vi "m10.wf.ramp.vi"(0 "Waveform In":waveform(dbl)={"t0"=timestamp(0 s since 1904-01-01), "dt"=0.0, "Y"=[]}, 5 "Ramp Length (s)":dbl=0.01, 11 "error in (no error)":errorcluster) -> (4 "Waveform Out":waveform(dbl), 15 "error out":errorcluster)   [LabVIEW 2013]
uses:
  <vilib>/Waveform/WDTOps.llb/WDT Waveform Duration DBL.vi
  <vilib>/Waveform/WDTOps.llb/WDT Append Waveforms DBL.vi
  <vilib>/measure/NI_MABase.lvlib
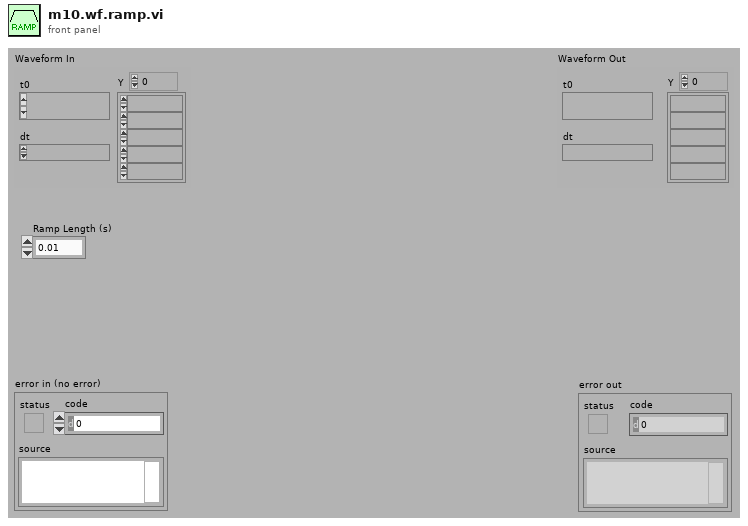
[diagram p1: front panel]
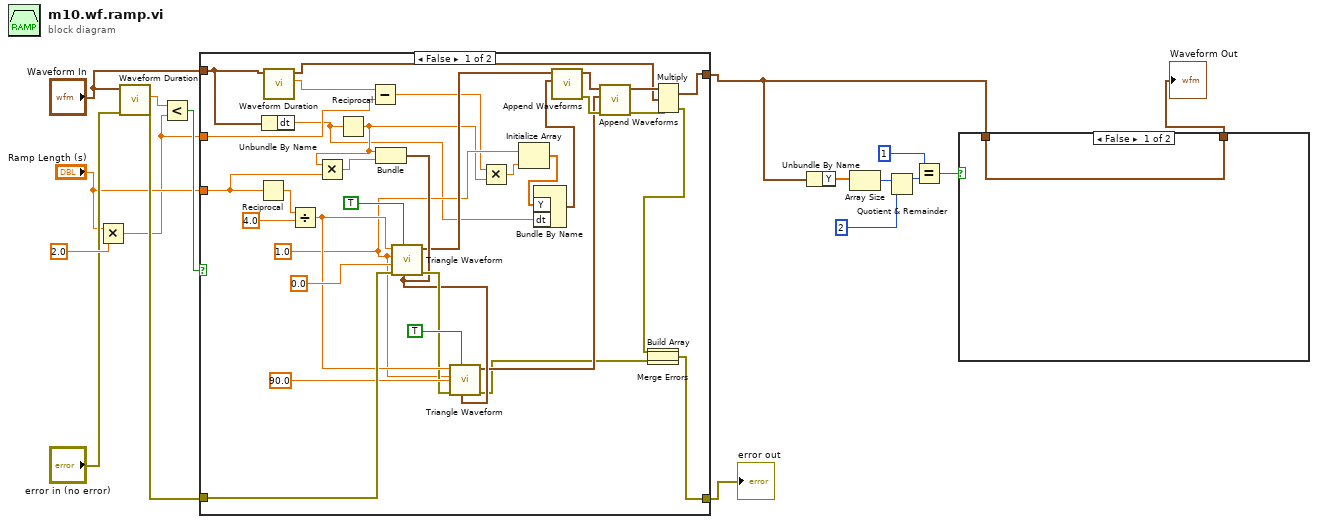
[diagram p0: block diagram]
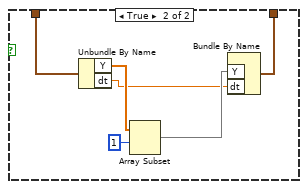
[diagram p2: hidden frame]
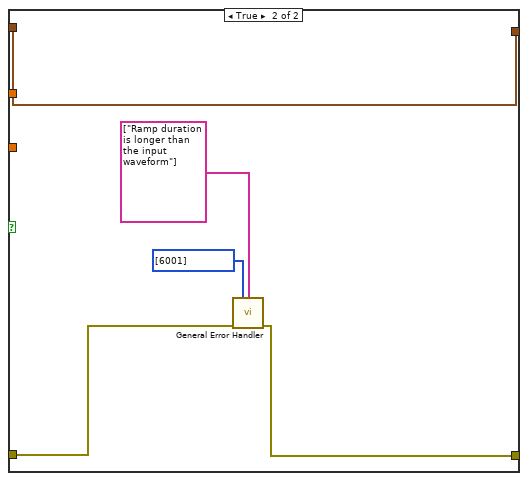
[diagram p3: hidden frame]
diagram:
  n1 = Multiply(x="Ramp Length (s)", y=2.0) -> (x*y=w9:dbl)
  n2 = call-poly <vilib>:"Waveform Duration.vi"("error in (no error)"="error in (no error)", "waveform in"="Waveform In") -> ("error out"=w13:errorcluster, "duration"=w17:dbl)  [unwired: 7 in, 1 out]
  n3 = Less?(x=w17, y=w9) -> (x < y?=w15:bool)
  n4 = case shown="False" w15 {
    tunnel: w13 -> [w48 w56]
    tunnel: [w26 w55] -> w11
    tunnel: "Waveform In" -> [w33 w52]
    tunnel: [w30 w52] -> w2
    tunnel: "Ramp Length (s)" -> [w36 _]
    tunnel: w9 -> [w34 _]
    frame False {
      w23 = 1.0 ("amplitude")
      n5 = Reciprocal(x=w36) -> (1/x=w51:dbl)
      n6 = Unbundle By Name(w33) -> ("dt"=w20:dbl)
      n7 = call-poly <vilib>:"Waveform Duration.vi"("waveform in"=w33) -> ("duration"=w31:dbl, "waveform out"=w32:waveform(dbl))  [unwired: 8 in, 1 out]
      n8 = Divide(x=w51, y=4.0) -> (x/y=w44:dbl)
      n9 = Reciprocal(x=w20) -> (1/x=w21:dbl)
      n10 = Multiply(x=w21, y=w36) -> (x*y=w47:dbl)
      n11 = Subtract(x=w31, y=w34) -> (x-y=w22:dbl)
      n12 = Bundle(w21, w47) -> (w41:cluster{dbl, dbl})  [unwired: 1 in]
      n13 = call <vilib>:"Triangle Waveform.vi"("sampling info"=w41, "reset signal"=TRUE, "error in (no error)"=w48, "phase"=0.0, "amplitude"=w23, "frequency"=w44) -> ("error out"=w42:errorcluster, "signal out"=w39:waveform(dbl))  [unwired: 4 in]
      n14 = call <vilib>:"Triangle Waveform.vi"("sampling info"=w41, "reset signal"=TRUE, "error in (no error)"=w42, "phase"=90.0, "amplitude"=w23, "frequency"=w44) -> ("error out"=w27:errorcluster, "signal out"=w37:waveform(dbl))  [unwired: 4 in]
      n15 = Multiply(x=w22, y=w21) -> (x*y=w24:dbl)
      n16 = Initialize Array(w23, w24) -> (w25:dbl[])
      n17 = Bundle By Name("Y"=w25, "dt"=w20) -> (w19:waveform(dbl))  [unwired: 1 in]
      n18 = call-poly <vilib>:"Append Waveforms.vi"("waveform B"=w19, "waveform A"=w39) -> ("error out"=w38:errorcluster, "waveform out"=w40:waveform(dbl))  [unwired: 8 in]
      n19 = call-poly <vilib>:"Append Waveforms.vi"("error in (no error)"=w38, "waveform B"=w37, "waveform A"=w40) -> ("error out"=w29:errorcluster, "waveform out"=w35:waveform(dbl))  [unwired: 7 in]
      n20 = Multiply(1:w32, 2:w35, 4:w29) -> (0:w30:waveform(dbl), 3:w28:errorcluster)
      n21 = Build Array(w28, w27) -> (w18:errorcluster[])
      n22 = Merge Errors(w18) -> (w26:errorcluster)
    }
    frame True {
      n23 = call <vilib>:"General Error Handler.vi"("[user-defined codes]"=i32[] [6001], "[user-defined descriptions]"=string[] ["Ramp duration is longer than the input waveform"], "error in (no error)"=w56) -> ("error out"=w55:errorcluster)  [unwired: 8 in, 4 out]
    }
  }
  "error out" <- w11
  n24 = Unbundle By Name(w2) -> ("Y"=w8:dbl[])
  n25 = Array Size(array=w8) -> (size(s)=w7:i32)
  n26 = Quotient & Remainder(x=w7, y=2) -> (x-y*floor(x/y)=w5:i32)  [unwired: 1 out]
  n27 = Equal?(x=1, y=w5) -> (x = y?=w3:bool)
  n28 = case shown="False" w3 {
    tunnel: w2 -> [w57 w63]
    tunnel: [w57 w58] -> w1
    frame False {
    }
    frame True {
      n29 = Unbundle By Name(w63) -> ("Y"=w62:dbl[], "dt"=w59:dbl)
      n30 = Array Subset(array=w62, index=1) -> (w60:dbl[])  [unwired: 1 in]
      n31 = Bundle By Name("Y"=w60, "dt"=w59) -> (w58:waveform(dbl))  [unwired: 1 in]
    }
  }
  "Waveform Out" <- w1
